vi "Draw_Region.vi"() -> ()   [LabVIEW 2010]
uses:
  gfitsio/gfitsio-read-image-subset-sgl-2d.vi
  <userlib>/gfitsio/gfitsio.lvlib
panel:
  out "calculating":bool
  out "ready":bool
  out "ZoomImg":sgl[][](graph)
  in  "stop":bool
  in  "n_sig":dbl
  out "variance":dbl format="%0.2f"
  out "median":dbl format="%0.2f"
  out "mean":dbl format="%0.2f"
  in  "lpixel (-1,-1: rest)":cluster{"X":i32, "Y":i32}={"X"=-1, "Y"=-1}
  in  "fpixel (1,1)":cluster{"X":i32, "Y":i32}={"X"=1, "Y"=1}
  out "header":string[](array[string])
  in  "path":path
  out "Intensity Graph":sgl[][](graph)
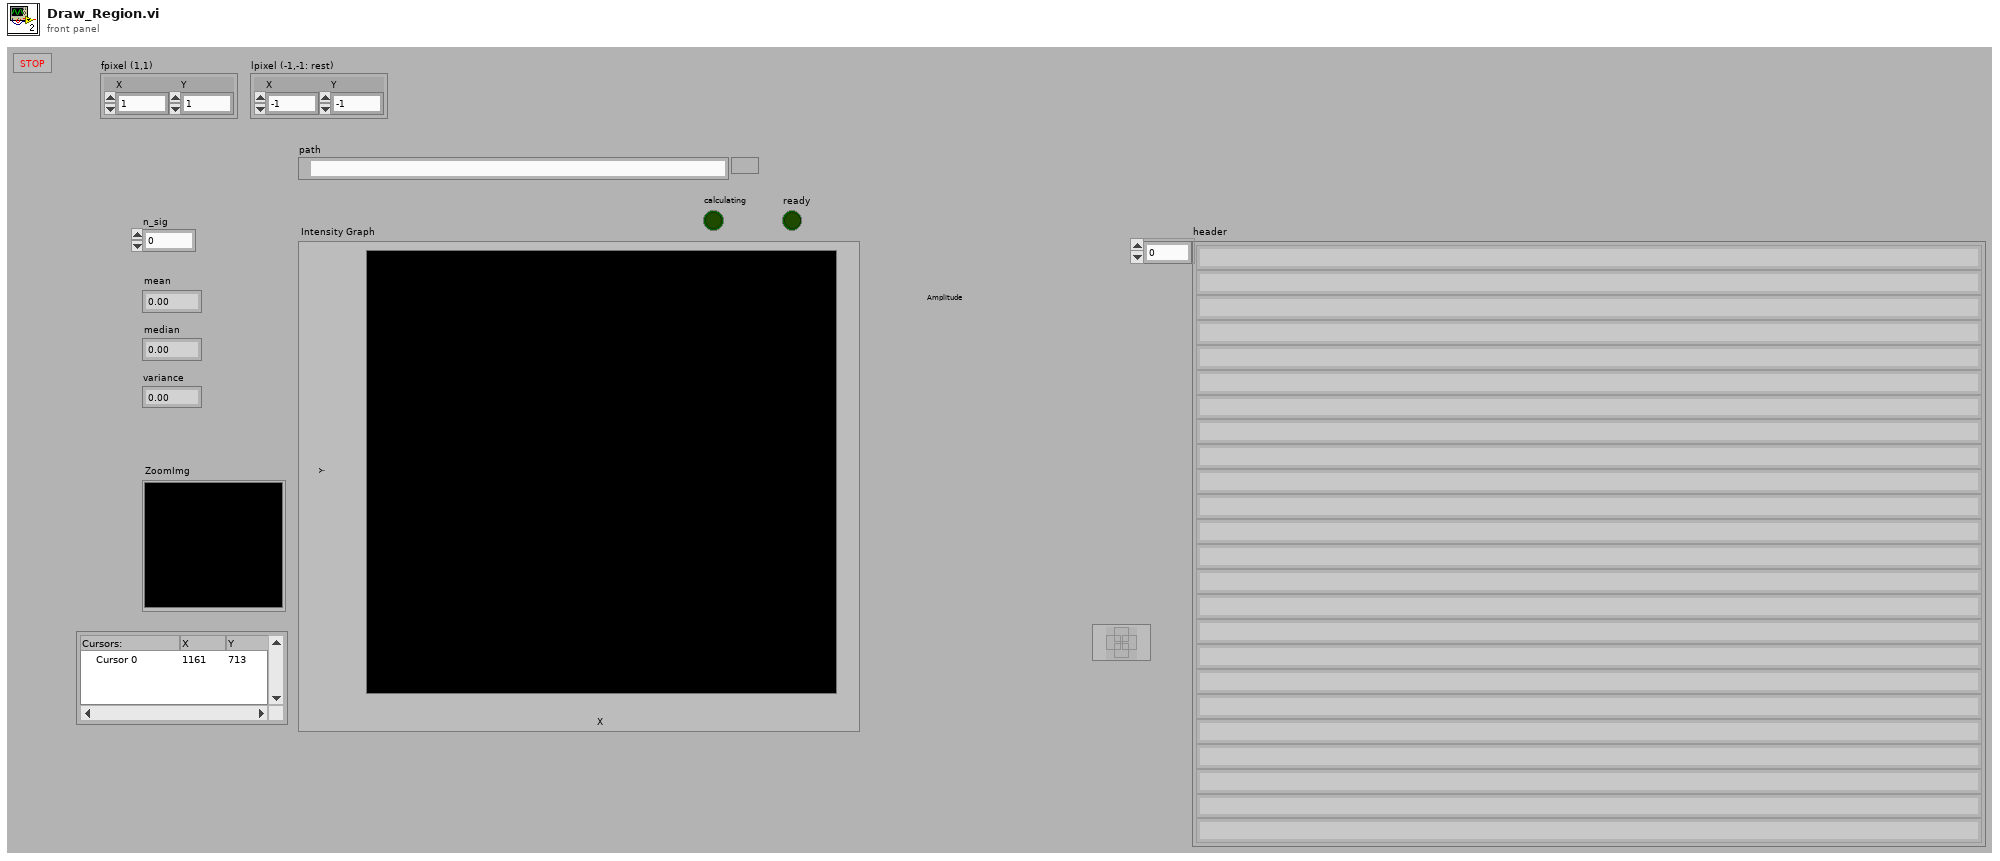
[diagram p1: front panel]
types:
  T1 = typedef "gfitsio.lvlib/gfitsio-refnum.ctl" = refnum<k1>
  T2 = cluster{"NAXIS":dbl[], "CD":dbl[][], "CDELT":dbl[], "CRPIX":dbl[], "CTYPE":string[], "CRVAL":dbl[], "LONGPOLE":dbl, "LATPOLE":dbl, "PV2":dbl[]}
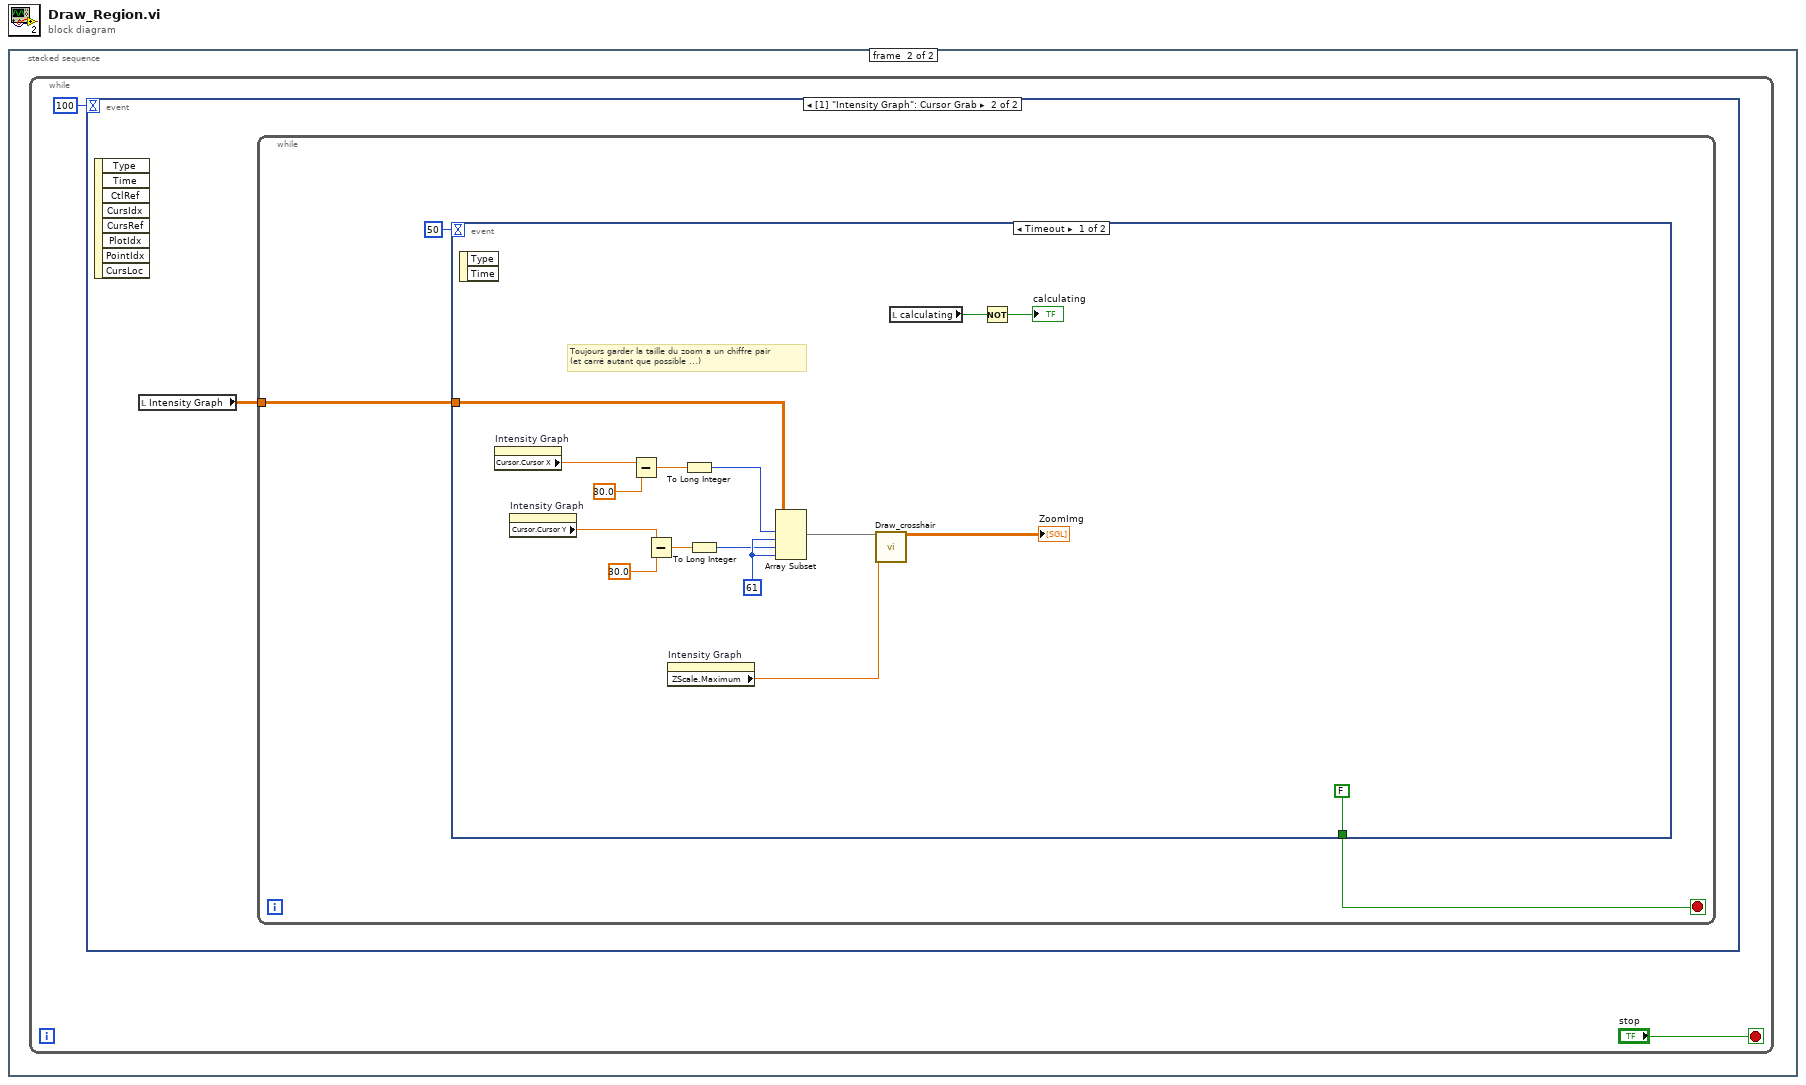
[diagram p0: block diagram]
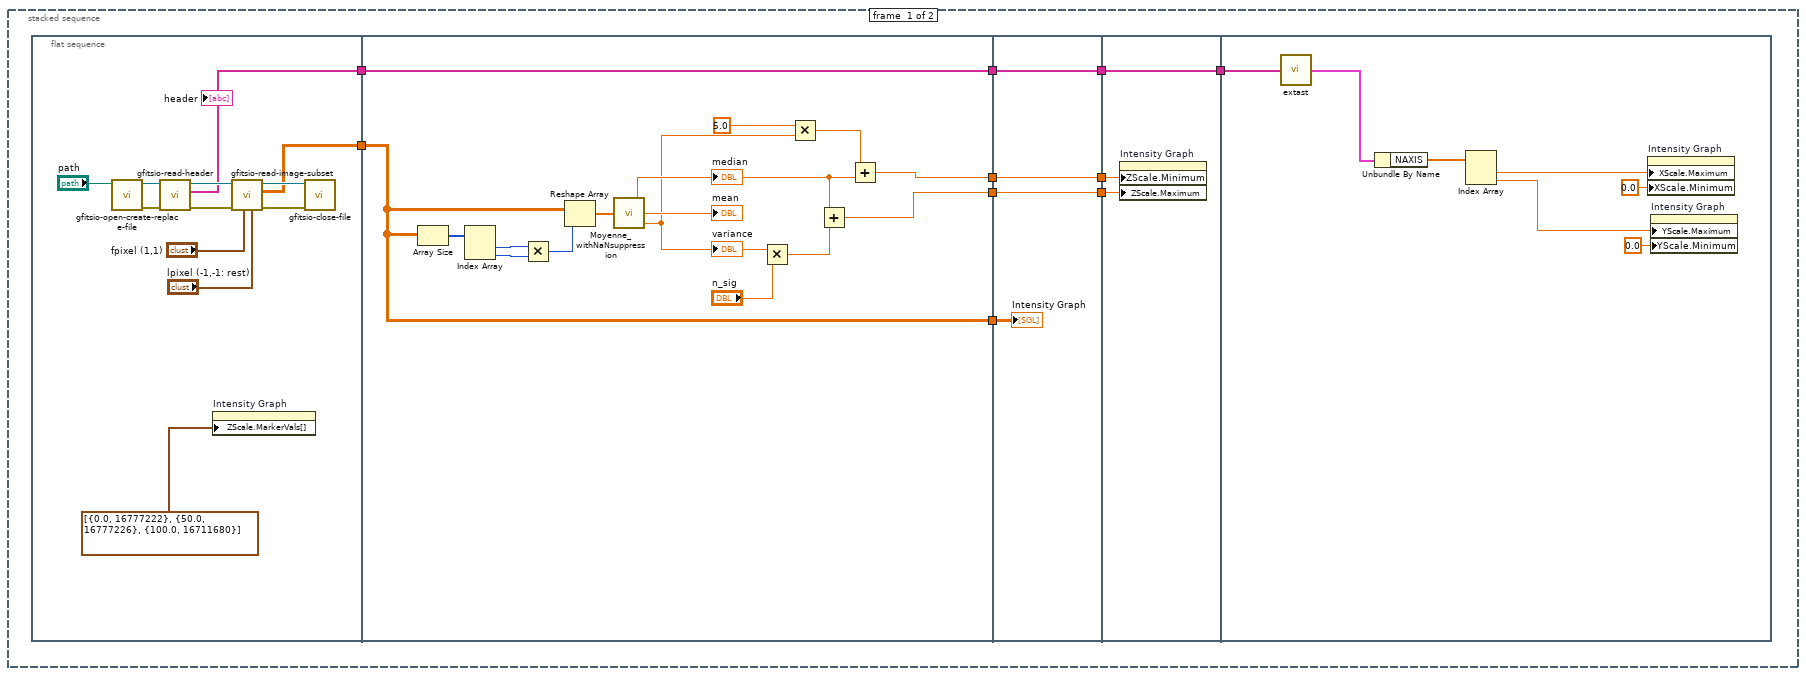
[diagram p2: hidden frame]
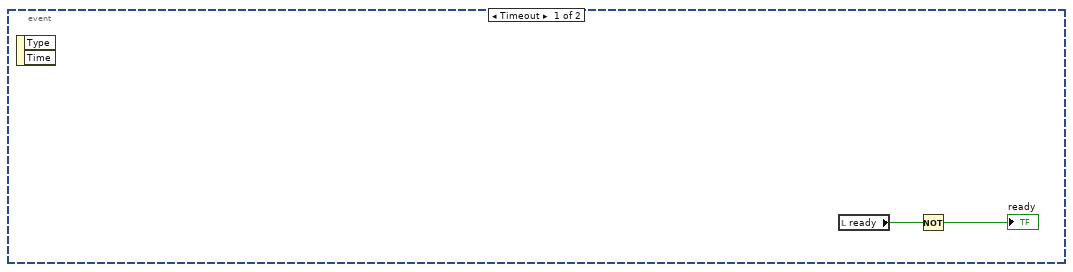
[diagram p3: hidden frame]
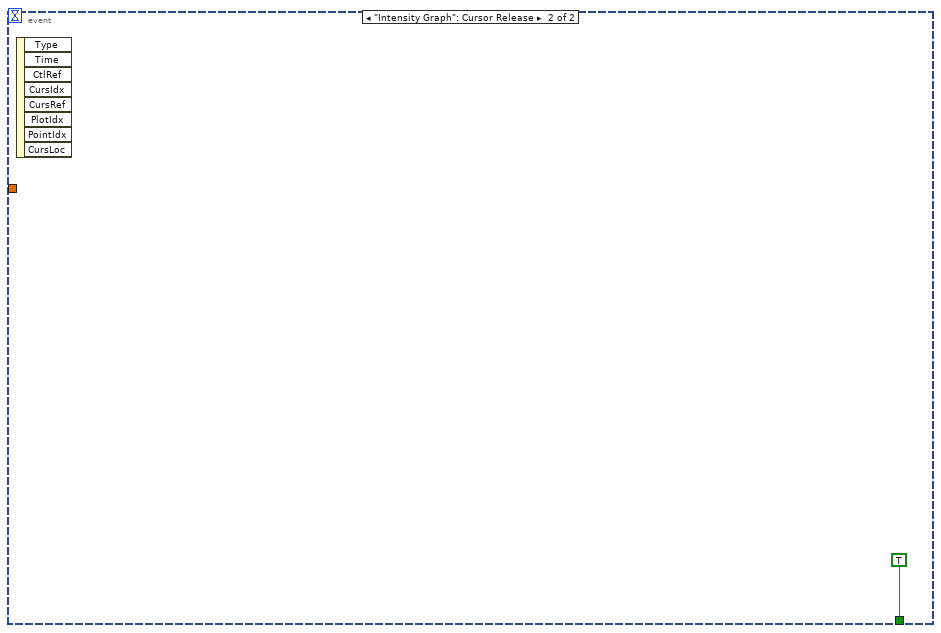
[diagram p4: hidden frame]
diagram:
  n1 = stacked-sequence {
    frame #0 {
      n2 = flat-sequence {
        tunnel: [w13] -> w10
        tunnel: [w12] -> w9
        tunnel: [w30] -> w8
        tunnel: w10 -> [w30]
        tunnel: w9 -> [w28]
        tunnel: [w26] -> w7
        tunnel: [w29] -> w6
        tunnel: [w28] -> w5
        tunnel: w8 -> [w39]
        tunnel: [w42] -> w4
        tunnel: w7 -> [w42]
        tunnel: [w41] -> w3
        tunnel: w6 -> [w41]
        tunnel: [w40] -> w2
        tunnel: w5 -> [w40]
        tunnel: w4 -> [w45]
        tunnel: w3 -> [w44]
        tunnel: w2 -> [w43]
        tunnel: [w43] -> w1
        tunnel: w1 -> [w52]
        frame #0 {
          n3 = call "gfitsio-open-create-replace-file.vi"("file path (dialog if empty)"="path") -> ("error out"=w18:errorcluster, "gfits refnum"=w17:T1)  [unwired: 8 in, 1 out]
          n4 = call "gfitsio-read-header.vi"("error in (no error)"=w18, "gfits refnum"=w17) -> ("error out"=w22:errorcluster, "header"=w12:string[], "dup gfits refnum"=w21:T1)  [unwired: 7 in]
          "header" <- w12
          n5 = property on="Intensity Graph" class="IntGraph (strict)"("ZScale.MarkerVals[]"=cluster{dbl, u32}[] [{0.0, 16777222}, {50.0, 16777226}, {100.0, 16711680}] ("Z Scale.Marker Values[]")) -> ()  [unwired: 2 in, 2 out]
          n6 = call-poly "gfitsio-read-image-subset.vi"("lpixel (-1,-1: rest)"="lpixel (-1,-1: rest)", "fpixel (1,1)"="fpixel (1,1)", "error in (no error)"=w22, "gfits refnum"=w21) -> ("error out"=w20:errorcluster, "data"=w13:sgl[][], "dup gfits refnum"=w19:T1)  [unwired: 4 in, 1 out]
          n7 = call "gfitsio-close-file.vi"("error in (no error)"=w20, "gfits refnum"=w19) -> ()  [unwired: 8 in, 2 out]
        }
        frame #1 {
          n8 = Array Size(array=w30) -> (size(s)=w36:i32[])
          n9 = Index Array(array=w36) -> (element #1=w35:i32, element #2=w34:i32)  [unwired: 2 in]
          n10 = Multiply(x=w35, y=w34) -> (x*y=w33:i32)
          n11 = Reshape Array(w30, w33) -> (w38:sgl[])
          n12 = call "Moyenne_withNaNsuppression.vi"("DBL-Array"=w38) -> ("Standard Deviation"=w24:dbl, "Average"=→"mean":dbl, "Median"=w27:dbl)  [unwired: 2 in]
          "median" <- w27
          "variance" <- w24
          n13 = Multiply(x=w24, y="n_sig") -> (x*y=w32:dbl)
          n14 = Multiply(x=5.0, y=w24) -> (x*y=w25:dbl)
          n15 = Add(x=w27, y=w32) -> (x+y=w29:dbl)
          n16 = Add(x=w25, y=w27) -> (x+y=w26:dbl)
        }
        frame #2 {
          "Intensity Graph" <- w39
        }
        frame #3 {
          n17 = property on="Intensity Graph" class="IntGraph (strict)"("ZScale.Minimum"=w45, "ZScale.Maximum"=w44) -> ()  [unwired: 2 in, 2 out]
        }
        frame #4 {
          n18 = call "extast.vi"("header"=w52) -> ("Astrometry"=w51:T2)  [unwired: 14 in]
          n19 = Unbundle By Name(w51) -> ("NAXIS"=w50:dbl[])
          n20 = Index Array(array=w50) -> (element #1=w49:dbl, element #2=w48:dbl)  [unwired: 2 in]
          n21 = property on="Intensity Graph" class="IntGraph (strict)"("XScale.Maximum"=w49, "XScale.Minimum"=0.0 ("X Scale.Range:Minimum")) -> ()  [unwired: 2 in, 2 out]
          n22 = property on="Intensity Graph" class="IntGraph (strict)"("YScale.Maximum"=w48, "YScale.Minimum"=0.0 ("Y Scale.Range:Minimum")) -> ()  [unwired: 2 in, 2 out]
        }
      }
    }
    frame #1 {
      n23 = while {
        stop <- "stop" stop-if-true
        n24 = event shown="[1] \"Intensity Graph\": Cursor Grab" {
          selector: _ -> [_ _]
          dyn-events: _ -> [_ _]
          timeout: 100 -> [_ _]
          event Timeout {
            n25 = event-data() -> ()  [unwired: 1 in, 2 out]
            n26 = local read "ready"() -> (w56:bool)
            n27 = Not(x=w56) -> (.not. x?=→"ready":bool)
          }
          event "Intensity Graph": Cursor Grab {
            n28 = event-data() -> ()  [unwired: 1 in, 8 out]
            n29 = local read "Intensity Graph"() -> (w57:sgl[][])
            n30 = while {
              tunnel: w57 -> [w60]
              stop <- w59 stop-if-true
              n31 = event shown="[0] Timeout" {
                selector: _ -> [_ _]
                dyn-events: _ -> [_ _]
                timeout: 50 -> [_ _]
                tunnel: w60 -> [w76 _]
                tunnel: [FALSE TRUE] -> w59
                event Timeout {
                  w68 = 61
                  # "Toujours garder la taille du zoom a un chiffre pair\n(et carré autant que possible ...)"
                  n32 = event-data() -> ()  [unwired: 1 in, 2 out]
                  n33 = property on="Intensity Graph" class="IntGraph (strict)"() -> ("Cursor.Cursor X"=w75:dbl)  [unwired: 2 in, 2 out]
                  n34 = property on="Intensity Graph" class="IntGraph (strict)"() -> ("Cursor.Cursor Y"=w71:dbl)  [unwired: 2 in, 2 out]
                  n35 = Subtract(x=w75, y=30.0) -> (x-y=w74:dbl)
                  n36 = Subtract(x=w71, y=30.0) -> (x-y=w69:dbl)
                  n37 = property on="Intensity Graph" class="IntGraph (strict)"() -> ("ZScale.Maximum"=w61:dbl)  [unwired: 2 in, 2 out]
                  n38 = To Long Integer(number=w74) -> (32bit integer=w70:i32)
                  n39 = To Long Integer(number=w69) -> (32bit integer=w67:i32)
                  n40 = Array Subset(array=w76, index (row)=w70, length (row)=w68, index (col)=w67, length (col)=w68) -> (w63:sgl[][])
                  n41 = call "Draw_crosshair.vi"("Image IN"=w63, "White Value"=w61) -> ("Image OUT"=→"ZoomImg":sgl[][])  [unwired: 13 in]
                  n42 = local read "calculating"() -> (w65:bool)
                  n43 = Not(x=w65) -> (.not. x?=→"calculating":bool)
                }
                event "Intensity Graph": Cursor Release {
                  n44 = event-data() -> ()  [unwired: 1 in, 8 out]
                }
              }
            }
          }
        }
      }
    }
  }
